vi "Get Map Cursor Offset.vi"(8 "error in (no error)":errorcluster, 11 "This VI":refnum<vi>) -> (0 "error out":errorcluster, 3 "Gmap Offset":T1)   [LabVIEW 2014]
uses:
  <vilib>/Utility/miscctls.llb/LVPositionTypeDef.ctl
panel:
  in  "GMap Position":T1
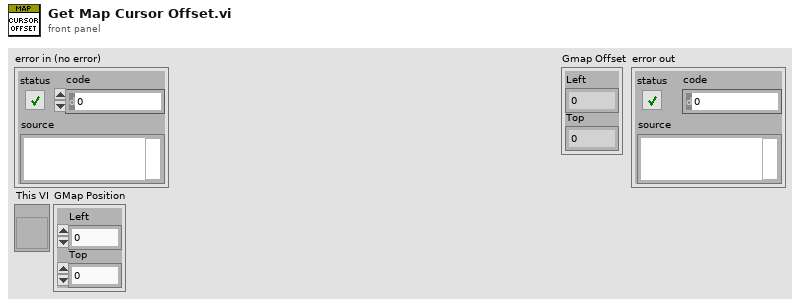
[diagram p1: front panel]
types:
  T1 = typedef "LVPositionTypeDef.ctl" = cluster{"Left":i32, "Top":i32}
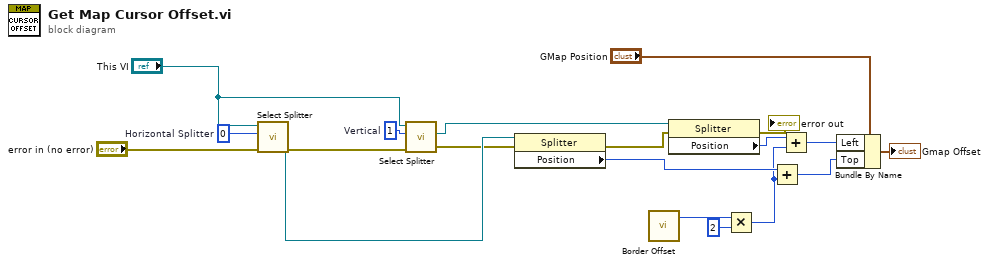
[diagram p0: block diagram]
diagram:
  w16 = 1  # Vertical
  w17 = 0  # Horizontal Splitter
  n1 = call "Select Splitter.vi"("error in (no error)"="error in (no error)", "Pane Index"=w17, "This VI"="This VI") -> ("error out"=w15:errorcluster, "Splitter"=w14:refnum<vi>)  [unwired: 6 in, 1 out]
  n2 = call "Select Splitter.vi"("error in (no error)"=w15, "Pane Index"=w16, "This VI"="This VI") -> ("error out"=w12:errorcluster, "Splitter"=w13:refnum<vi>)  [unwired: 6 in, 1 out]
  n3 = property class="Splitter"(reference=w14, error in=w12) -> (error out=w11:errorcluster, "Position"=w9:i32)  [unwired: 1 out]
  n4 = call "Border Offset.vi"() -> ("Border Offset (px)"=w3:i32)  [unwired: 11 in]
  n5 = property class="Splitter"(reference=w13, error in=w11) -> (error out=→"error out":errorcluster, "Position"=w7:i32)  [unwired: 1 out]
  n6 = Multiply(x=w3, y=2) -> (x*y=w1:i32)
  n7 = Add(x=w9, y=w1) -> (x+y=w8:i32)
  n8 = Add(x=w7, y=w1) -> (x+y=w6:i32)
  n9 = Bundle By Name(cluster="GMap Position", "Left"=w6, "Top"=w8) -> (→"Gmap Offset":T1)
